vi "TDMS Read Log Test Program.vi"() -> (2 "data 2":dbl[][](array[numeric]), 3 "data":timestamp[][](array[timestamp]), 11 "group/channel names":string[][](array[string]))   [LabVIEW 2020]
panel:
  in  "file path":path=path "C:/Users/gsfcprime/Documents/LabVIEW Data/TDMS/2021_239_01_Camera Control.tdms_index"
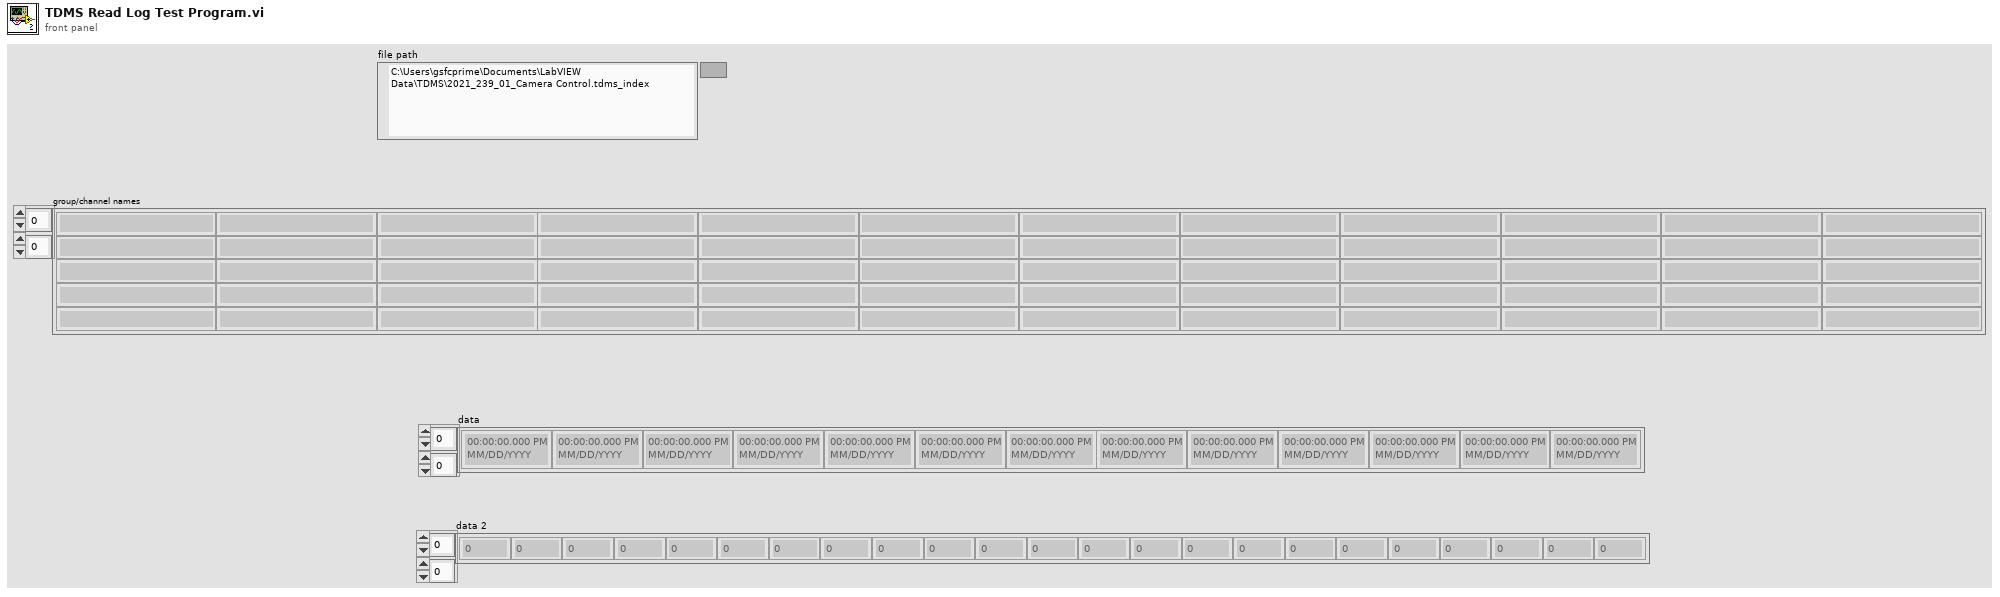
[diagram p1: front panel]
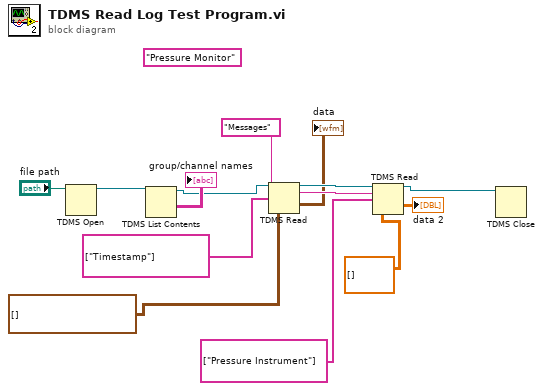
[diagram p0: block diagram]
diagram:
  (unwired) "Pressure Monitor" ("group name in")
  n1 = TDMS Open(11:"file path") -> (3:w14:refnum<k34>)  [unwired: 6 in, 1 out]
  n2 = TDMS List Contents(7:w14) -> (1:→"group/channel names":string[][], 3:w11:refnum<k34>)  [unwired: 2 in, 2 out]
  n3 = TDMS Read(0:w11, 5:"Messages" ("group name in"), 7:string[] ["Timestamp"] ("channel name(s) in"), 12:timestamp[][] []) -> (4:w8:refnum<k34>, 6:w5:string, 10:→"data":timestamp[][])  [unwired: 4 in, 3 out]
  n4 = TDMS Read(0:w8, 5:w5, 7:string[] ["Pressure Instrument"] ("channel name(s) in"), 12:dbl[][] []) -> (4:w7:refnum<k34>, 10:→"data 2":dbl[][])  [unwired: 4 in, 4 out]
  n5 = TDMS Close(11:w7) -> ()  [unwired: 1 in, 2 out]
